vi "GraphSetting Conv ScaleFit.vi"(11 "自動スケール?":bool) -> (3 "Xスケール.スケールフィット":u8)   [LabVIEW 2014]
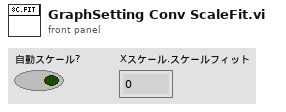
[diagram p1: front panel]
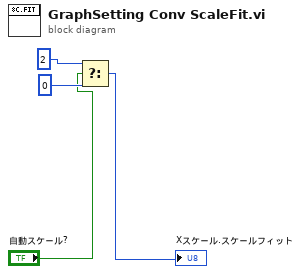
[diagram p0: block diagram]
diagram:
  n1 = Select(t=u8 2 ("Xスケール.スケールフィット"), s="自動スケール?", f=u8 0 ("Xスケール.スケールフィット")) -> (s? t:f=→"Xスケール.スケールフィット":u8)
